vi "ArmWithdraw.vi"() -> ()   [LabVIEW 2018]
panel:
  in  "ArmWithdraw":bool
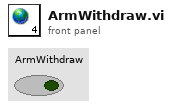
[diagram p1: front panel]
diagram:
